vi "GPIO Write Pull.vi"(7 "GPIO #":T1=-1, 8 "error in (no error)":errorcluster, 10 "GPIO Pull":T2, 11 "FirmwareComms in":refnum<class "VisaComms.lvclass">) -> (0 "error out":errorcluster, 3 "FirmwareComms out":refnum<class "VisaComms.lvclass">)   [LabVIEW 2024, in "CTI.lvlib" / "VisaComms.lvclass"]
uses:
  VisaComms.lvclass
  GPIO Pull.ctl
  GPIO Number.ctl
  VisaComms.lvclass/VisaComms.ctl
  Clean Visa Errors.vi
  CTI.lvlib
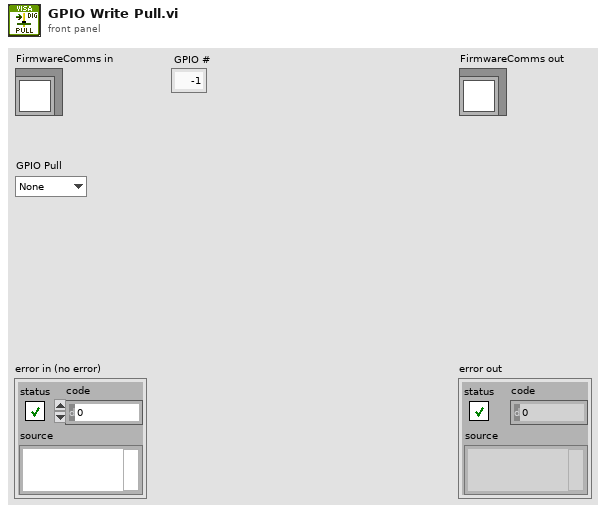
[diagram p1: front panel]
types:
  T1 = typedef "CTI.lvlib/GPIO Number.ctl" = i8
  T2 = typedef "CTI.lvlib/GPIO Pull.ctl" = enum16{"None", "Up", "Down", "Both"}
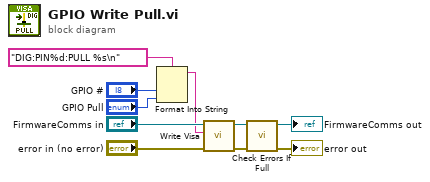
[diagram p0: block diagram]
diagram:
  n1 = Format Into String(format string="DIG:PIN%d:PULL %s\n", "GPIO #", "GPIO Pull") -> (resulting string=w4:string)  [unwired: 2 in, 1 out]
  n2 = call "Write Visa.vi"("error in (no error)"="error in (no error)", "write buffer"=w4, "VisaComms in"="FirmwareComms in") -> ("error out"=w2:errorcluster, "VisaComms out"=w6:refnum<class "VisaComms.lvclass">)  [unwired: 6 in, 1 out]
  n3 = call "Check Errors If Full.vi"("error in (no error)"=w2, "VisaComms in"=w6) -> ("error out"=→"error out":errorcluster, "VisaComms out"=→"FirmwareComms out":refnum<class "VisaComms.lvclass">)  [unwired: 8 in]
